vi "ABB SaveXYGraphImage_JPEG.vi"(2 "Path":path, 3 "COntrolReference":refnum<vi>) -> ()   [LabVIEW 2017]
panel:
  out "Picture":picture
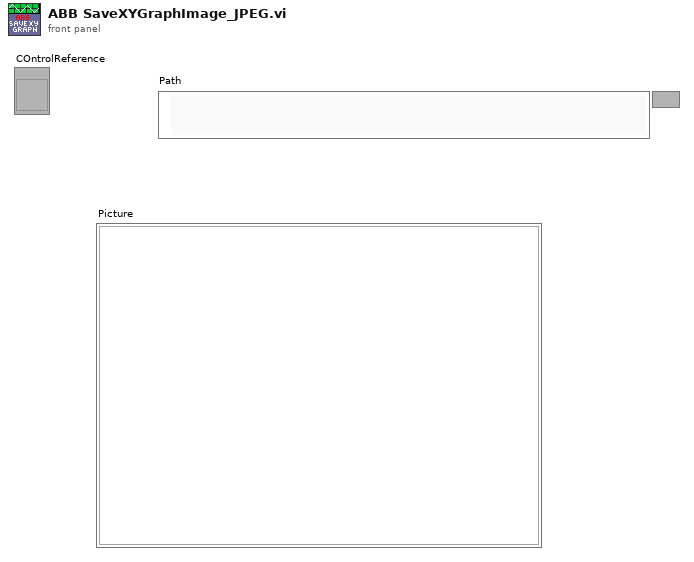
[diagram p1: front panel]
types:
  T1 = typedef "imagedata.ctl" = cluster{"image type":i32, "image depth":i32, "image":u8[], "mask":u8[], "colors":u32[], "Rectangle":cluster{"left":i16, "top":i16, "right":i16, "bottom":i16}}
  T2 = cluster{"left":i16, "top":i16, "right":i16, "bottom":i16}
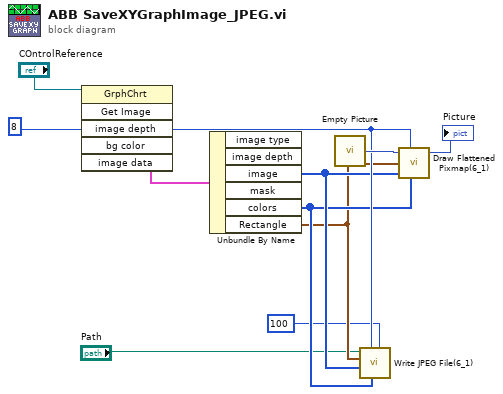
[diagram p0: block diagram]
diagram:
  w8 = 8 ("image depth")
  n1 = invoke class="GrphChrt" method="Get Image"(reference="COntrolReference") -> ("image data"=w7:T1)  [unwired: 5 in, 5 out]
  n2 = Unbundle By Name(w7) -> ("image"=w6:u8[], "colors"=w5:u32[], "Rectangle"=w4:T2)  [unwired: 3 out]
  n3 = call "Empty Picture"() -> ("empty picture"=w9:picture)
  n4 = call <vilib>:"Write JPEG File(6_1).vi"("quality (80)"=100, "color table"=w5, "depth"=w8, "flattened image data"=w6, "rect"=w4, "path to JPEG file"="Path") -> ()  [unwired: 4 in, 2 out]
  n5 = call <vilib>:"Draw Flattened Pixmap(6_1).vi"("picture"=w9, "bit depth(8)"=w8, "rect"=w4, "flattened pixmap data"=w6, "color table"=w5) -> ("new picture"=→"Picture":picture)  [unwired: 4 in]
